vi "SRV_PM_Unstuff.vi"(0 "Stuffed Data":u8[](array[numeric]) format="%.0x", 11 "error in (no error)":errorcluster) -> (4 "Stuffed Data dup":u8[](array[numeric]) format="%.0x", 8 "Data":u8[](array[numeric]) format="%.0x", 14 "Remaining Stuffed Data":u8[](array[numeric]) format="%.0x", 15 "error out":errorcluster)   [LabVIEW 2009]
uses:
  SRV_PM_Packet.ctl
panel:
  in  "Stuffing Byte (0x00)":u8 format="%.0x"
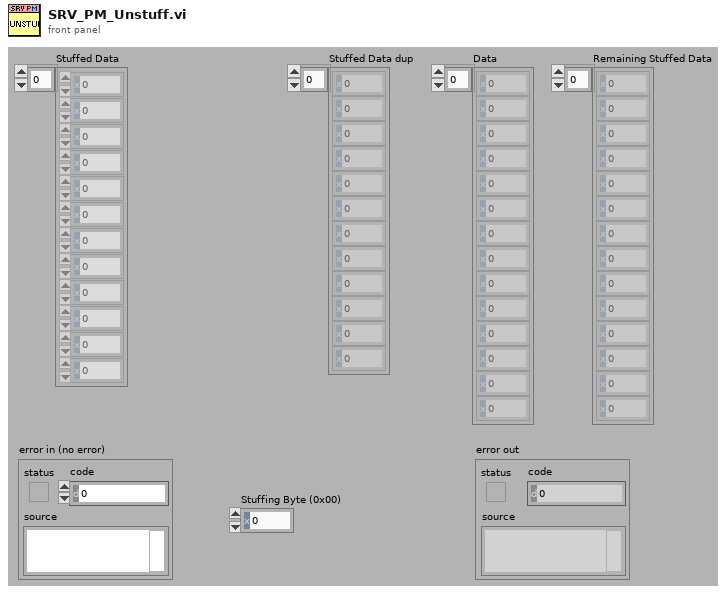
[diagram p1: front panel]
types:
  T1 = typedef "SRV_PM_Packet.ctl" = cluster{"Packet Data":u8[], "Complete?":bool, "Error?":bool}
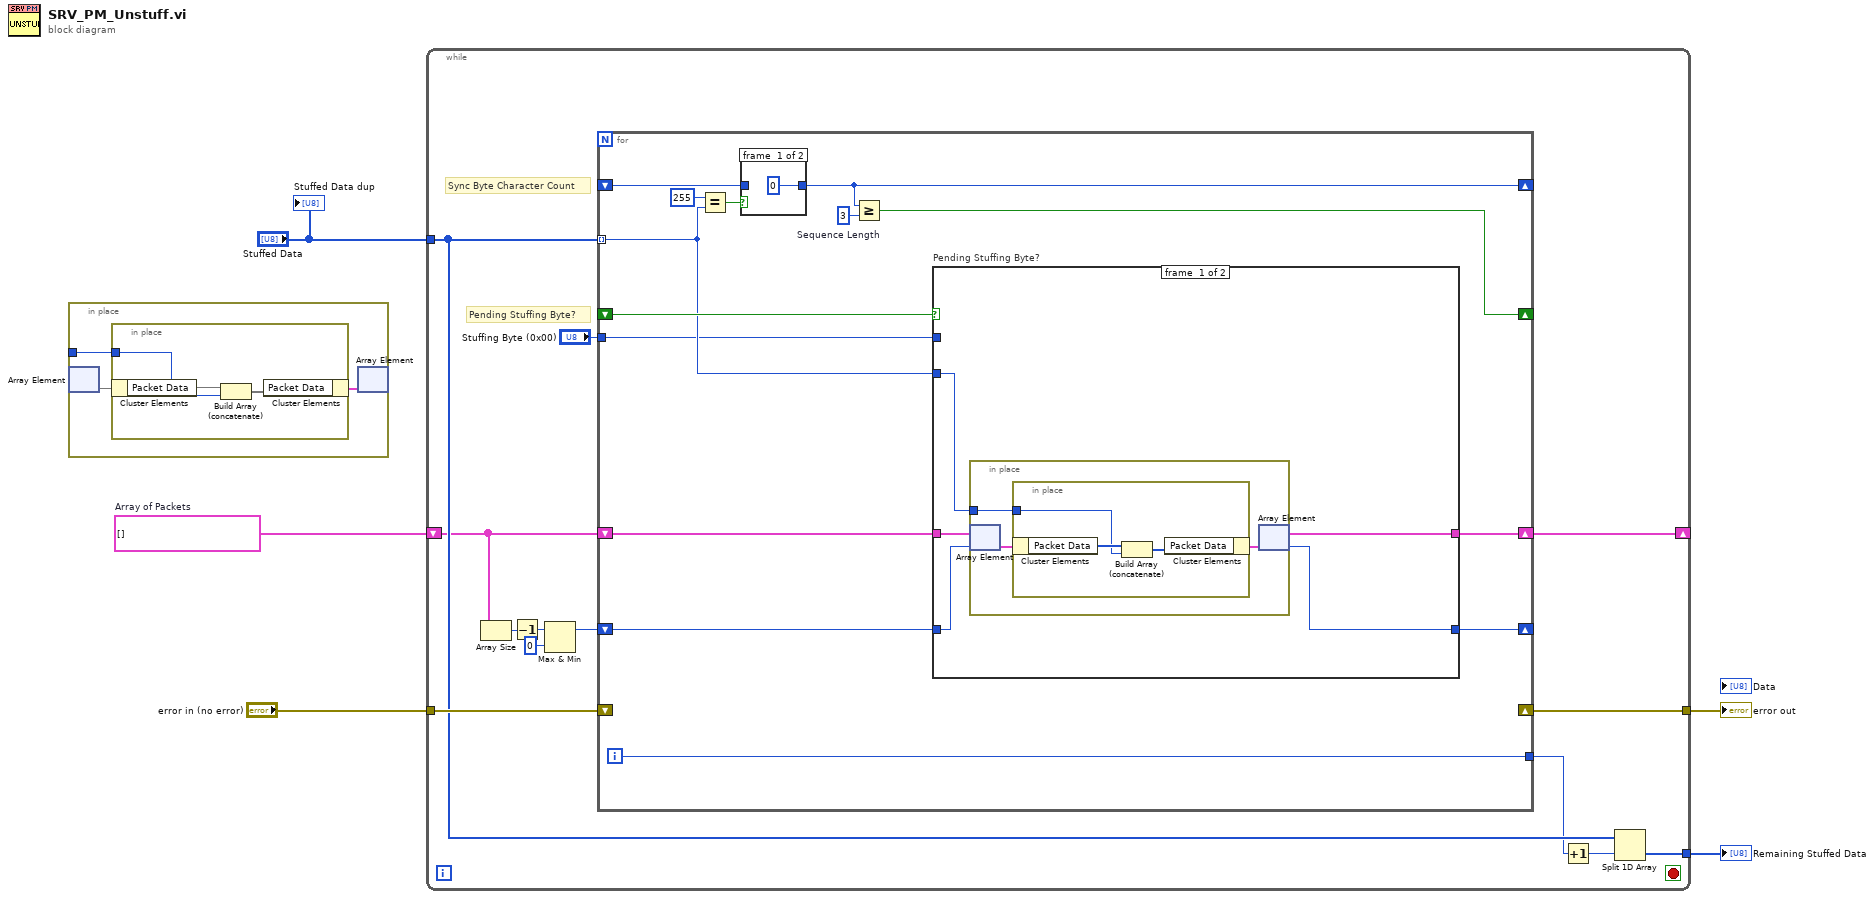
[diagram p0: block diagram]
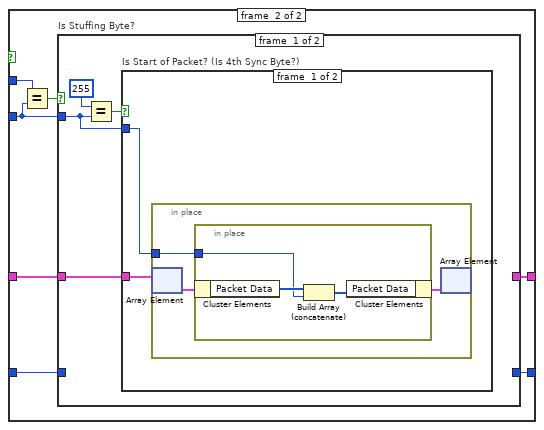
[diagram p2: hidden frame]
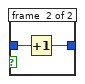
[diagram p5: hidden frame]
diagram:
  w1 = T1[] []  # Array of Packets
  n1 = in-place {
    in-place-border: _ -> [w7]
    n2 = in-place-array #1() -> (w8)  [unwired: 2 in]
    n3 = in-place {
      in-place-border: w7 -> [w10]
      n4 = in-place-cluster #2(w8) -> ("Packet Data"=w11)
      n5 = Build Array (concatenate)(w11, w10) -> (w9:void[])
      n6 = in-place-cluster #2("Packet Data"=w9) -> (w6:cluster{})
    }
    n7 = in-place-array #1(w6) -> ()  [unwired: 2 out]
  }
  n8 = while {
    tunnel: "error in (no error)" -> [w23]
    tunnel: [w22] -> w4
    tunnel: "Stuffed Data" -> [w21]
    tunnel: [w20] -> w2
    shift-right: [w12] -> _
    shift-left: w1 -> [w13]
    stop <- _ stop-if-true
    # "Pending Stuffing Byte?"
    # "Sync Byte Character Count"
    n9 = Array Size(array=w13) -> (size(s)=w17:i32)
    n10 = Decrement(x=w17) -> (x-1=w16:i32)
    n11 = Max & Min(x=w16, y=0) -> (max(x,y)=w14:i32)  [unwired: 1 out]
    n12 = for {
      tunnel: w21 -> [w31] mode=indexing
      tunnel: "Stuffing Byte (0x00)" -> [w30]
      shift-right: [_] -> w22
      shift-left: w23 -> [_]
      tunnel: [w38] -> w19
      shift-right: [w34] -> _
      shift-left: _ -> [w36]
      shift-right: [w33] -> _
      shift-left: _ -> [w32]
      shift-right: [w26] -> _
      shift-left: w14 -> [w27]
      shift-right: [w25] -> w12
      shift-left: w13 -> [w28]
      i -> [w38]
      w35 = 3  # Sequence Length
      n13 = Equal?(x=u8 255, y=w31) -> (x = y?=w37:bool)
      n14 = case shown="True" w37 {
        tunnel: w36 -> [_ w73]
        tunnel: [0 w72] -> w34
        frame #0 {
        }
        frame #1 {
          n15 = Increment(x=w73) -> (x+1=w72:i32)
        }
      }
      n16 = Greater Or Equal?(x=w34, y=w35) -> (x >= y?=w33:bool)
      n17 = case "Pending Stuffing Byte?" shown="True" w32 {
        tunnel: w31 -> [w42 w50]
        tunnel: w30 -> [_ w56]
        tunnel: w28 -> [w43 w54]
        tunnel: w27 -> [w41 w52]
        tunnel: [w40 w51] -> w26
        tunnel: [w39 w53] -> w25
        frame #0 {
          n18 = in-place {
            in-place-border: w42 -> [w45]
            n19 = in-place-array #3(w43, w41) -> (w46:T1)
            n20 = in-place {
              in-place-border: w45 -> [w48]
              n21 = in-place-cluster #4(w46) -> ("Packet Data"=w49:u8[])
              n22 = Build Array (concatenate)(w49, w48) -> (w47:u8[])
              n23 = in-place-cluster #4("Packet Data"=w47) -> (w44:T1)
            }
            n24 = in-place-array #3(w44) -> (w39:T1[], w40:i32)
          }
        }
        frame #1 {
          n25 = Equal?(x=w56, y=w50) -> (x = y?=w55:bool)
          n26 = case "Is Stuffing Byte?" shown="False" w55 {
            tunnel: w50 -> [w59 _]
            tunnel: w54 -> [w57 w70]
            tunnel: [_ w70] -> w53
            tunnel: w52 -> [_ w69]
            tunnel: [_ w69] -> w51
            frame #0 {
              n27 = Equal?(x=u8 255, y=w59) -> (x = y?=w60:bool)
              n28 = case "Is Start of Packet? (Is 4th Sync Byte?)" shown="True" w60 {
                tunnel: w59 -> [w61 _]
                tunnel: w57 -> [w62 _]
                frame #0 {
                  n29 = in-place {
                    in-place-border: w61 -> [w64]
                    n30 = in-place-array #5(w62) -> (w65:T1)  [unwired: 1 in]
                    n31 = in-place {
                      in-place-border: w64 -> [w67]
                      n32 = in-place-cluster #6(w65) -> ("Packet Data"=w68:u8[])
                      n33 = Build Array (concatenate)(w68, w67) -> (w66:u8[])
                      n34 = in-place-cluster #6("Packet Data"=w66) -> (w63:T1)
                    }
                    n35 = in-place-array #5(w63) -> ()  [unwired: 2 out]
                  }
                }
                frame #1 {
                }
              }
            }
            frame #1 {
            }
          }
        }
      }
    }
    n36 = Increment(x=w19) -> (x+1=w18:i32)
    n37 = Split 1D Array(array=w21, index=w18) -> (second subarray=w20:u8[])  [unwired: 1 out]
  }
  "error out" <- w4
  "Remaining Stuffed Data" <- w2
  "Stuffed Data dup" <- "Stuffed Data"
